vi "pythonHyperstackTest2.vi"() -> ()   [LabVIEW 2017]
uses:
  globalUtilities.vi
panel:
  out "Numeric":i32
  out "optogGUIX":dbl
  out "optogGUIY":dbl
  out "optogGUIZ":dbl
  in  "stop":bool
  # "Arrays work only if they have size >1 (2 is fine). Dunno why."
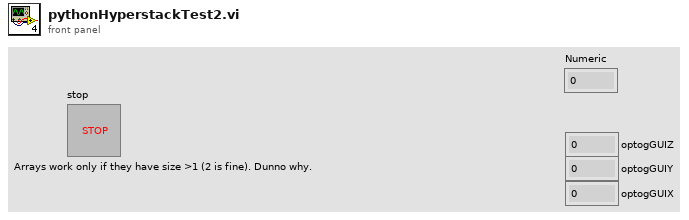
[diagram p1: front panel]
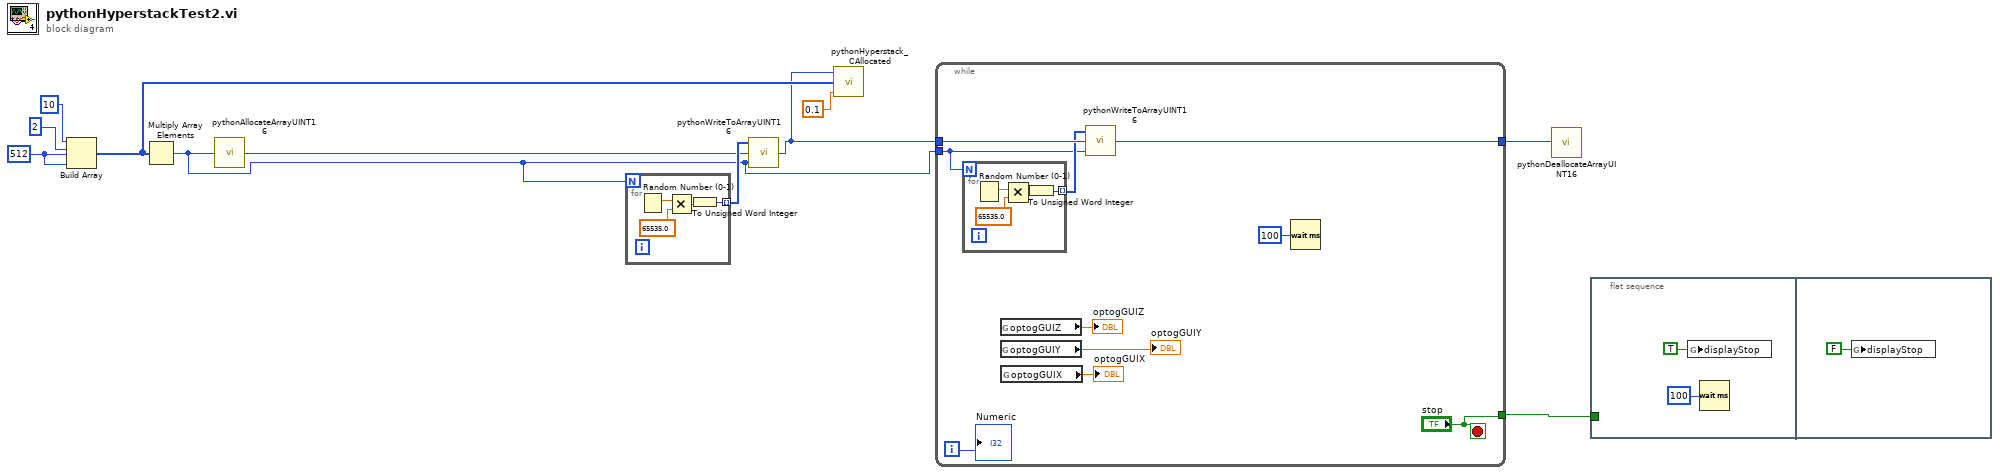
[diagram p0: block diagram]
diagram:
  w2 = 512 ("element")
  n1 = Build Array(10 ("element"), 2 ("element"), w2, w2) -> (w6:i32[])
  n2 = Multiply Array Elements(1:w6) -> (0:w8:i32)
  n3 = call "pythonAllocateArrayUINT16.vi"("size"=w8) -> ("pointer"=w5:i64)
  n4 = for {
    N: w8 -> [_]
    tunnel: [w15] -> w9 mode=indexing
    n5 = Random Number (0-1)() -> (number: 0 to 1=w14:dbl)
    n6 = Multiply(x=w14, y=65535.0) -> (x*y=w12:dbl)
    n7 = To Unsigned Word Integer(number=w12) -> (unsigned 16bit integer=w15:u16)
  }
  n8 = call "pythonWriteToArrayUINT16.vi"("size"=w8, "dst"=w5, "src"=w9) -> ("dst out"=w1:i64)
  n9 = call "pythonHyperstack_CAllocated.vi"("refresh_time"=0.1, "shape"=w6, "ptr"=w1) -> ()  [unwired: 1 out]
  n10 = while {
    tunnel: ["stop"] -> w11
    tunnel: w1 -> [w21]
    tunnel: w8 -> [w16]
    tunnel: [w20] -> w10
    i -> [w19]
    stop <- "stop" stop-if-true
    n11 = for {
      N: w16 -> [_]
      tunnel: [w29] -> w18 mode=indexing
      n12 = Random Number (0-1)() -> (number: 0 to 1=w28:dbl)
      n13 = Multiply(x=w28, y=65535.0) -> (x*y=w26:dbl)
      n14 = To Unsigned Word Integer(number=w26) -> (unsigned 16bit integer=w29:u16)
    }
    n15 = global read "globalUtilities.vi" "optogGUIZ"() -> (→"optogGUIZ":dbl)
    n16 = global read "globalUtilities.vi" "optogGUIY"() -> (→"optogGUIY":dbl)
    n17 = global read "globalUtilities.vi" "optogGUIX"() -> (→"optogGUIX":dbl)
    n18 = call "pythonWriteToArrayUINT16.vi"("size"=w16, "dst"=w21, "src"=w18) -> ("dst out"=w20:i64)
    n19 = Wait (ms)(milliseconds to wait=u32 100) -> ()  [unwired: 1 out]
    "Numeric" <- w19
  }
  n20 = call "pythonDeallocateArrayUINT16.vi"("ptr"=w10) -> ()  [unwired: 1 in]
  n21 = flat-sequence {
    tunnel: w11 -> [_]
    frame #0 {
      n22 = global write "globalUtilities.vi" "displayStop"(TRUE ("generalStop")) -> ()
      n23 = Wait (ms)(milliseconds to wait=u32 100) -> ()  [unwired: 1 out]
    }
    frame #1 {
      n24 = global write "globalUtilities.vi" "displayStop"(FALSE ("generalStop")) -> ()
    }
  }
